vi "绘制识别区.vi"(8 "error in (no error)":errorcluster, 9 "内框":T3(array[cluster]), 10 "外框":T1={"Left"=8, "Top"=43, "Right"=632, "Bottom"=436}, 11 "Image":T2) -> (0 "error out":errorcluster, 3 "Image Out":T2)   [LabVIEW 2018]
uses:
  <vilib>/vision/Image Controls.llb/IMAQ Image.ctl
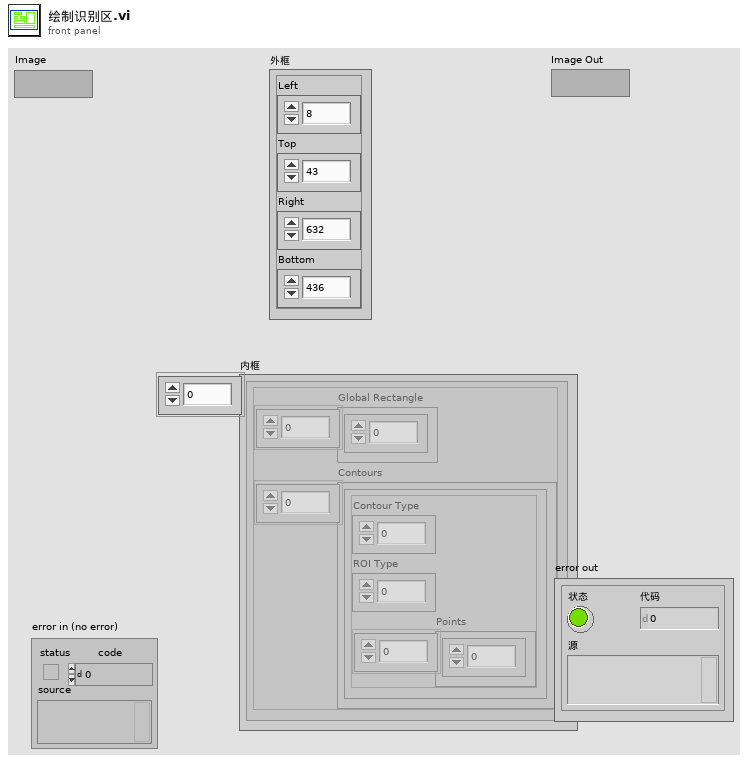
[diagram p1: front panel]
types:
  T1 = cluster{"Left":i32, "Top":i32, "Right":i32, "Bottom":i32}
  T2 = typedef "IMAQ Image.ctl" = refnum<image>
  T3 = cluster{"Global Rectangle":i32[], "Contours":cluster{"Contour Type":u32, "ROI Type":u32, "Points":i32[]}[]}[]
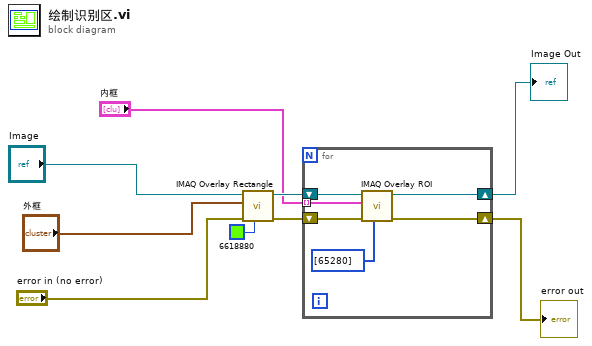
[diagram p0: block diagram]
diagram:
  n1 = call "IMAQ Overlay Rectangle"("Color"=u32 6618880, "error in (no error)"="error in (no error)", "Rectangle"="外框", "Image"="Image") -> ("error out"=w3:errorcluster, "Image Out"=w5:T2)  [unwired: 6 in]
  n2 = for {
    tunnel: "内框" -> [w14] mode=indexing
    shift-right: [w11] -> w1
    shift-left: w3 -> [w12]
    shift-right: [w10] -> w2
    shift-left: w5 -> [w15]
    n3 = call "IMAQ Overlay ROI"("Colors (Green)"=u32[] [65280], "error in (no error)"=w12, "ROI Descriptor"=w14, "Image"=w15) -> ("error out"=w11:errorcluster, "Image Out"=w10:T2)  [unwired: 6 in]
  }
  "Image Out" <- w2
  "error out" <- w1
